vi "Camer Control Main.vi"() -> ()   [LabVIEW 2014]
uses:
  <vilib>/MakerHub/LINX/Public/Utilities/Open Local.vi
  FGV/Camer Control Variables.vi
  Application Support/Stop Button/SubVI/Get Stop Button Status.vi
  Aircraft Information/Sub VI/Get Aircraft Information.vi
  <vilib>/MakerHub/LINX/LMH-LINX.lvlib
panel:
  out "Device Name":string
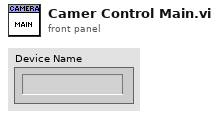
[diagram p1: front panel]
types:
  T1 = typedef "LMH-LINX.lvlib/LINX Ref.ctl" = cluster{"IO":T2, "Interface":T3, "LINX Device Config":T4}
  T2 = typedef "LMH-LINX.lvlib/Platform.ctl" = enum16{"Remote", "Local"}
  T3 = typedef "LMH-LINX.lvlib/Interface.ctl" = enum16{"Serial", "TCP"}
  T4 = typedef "LMH-LINX.lvlib/Device.lvlib/LINX Device Config.ctl" = cluster{"Interface":T3, "COM Port":refnum<visa-resource-name>, "TCP Configuration":T5, "Device Family":u8, "Device ID":u8, "Device Name":string, "TCP Ref":refnum<k5>, "Channels":T6}
  T5 = typedef "LMH-LINX.lvlib/Device.lvlib/TCP Config.ctl" = cluster{"IP Address":string, "Port":u16}
  T6 = typedef "LMH-LINX.lvlib/Channels.ctl" = cluster{"DI":u8[], "DO":u8[], "AI":u8[], "AO":u8[], "PWM":u8[], "QE":u8[], "UART":u8[], "I2C 2":u8[], "SPI":u8[], "CAN":u8[], "Servo":u8[], "AI Ref (V)":dbl, "AI Resolution (Bits)":u8, "AO Ref (V)":dbl, "AO Resolution (Bits)":u8}
  T7 = typedef "Drone Information.ctl" = cluster{"Aircraft ID":u8, "Tag ID":string, "System Status":string, "Base Mode":T8, "Armed/Disarmed":bool, "Battery Voltage":dbl, "Control Mode":T9, "Initialisation":u8, "Coms with aircraft good":bool, "Mode":string, "Mission Uploaded":bool}
  T8 = typedef "Base Mode.ctl" = cluster{"Custom Mode":bool, "Test Enabled":bool, "Autonomous Mode":bool, "Guided Mode":bool, "Stabilization Enabled":bool, "HIL Enabled":bool, "Manual Mode":bool, "Arm":bool}
  T9 = typedef "Aircraft Mode.ctl" = enum16{"Loiter", "Stabalise", "Failsafe", "Emergency Stop"}
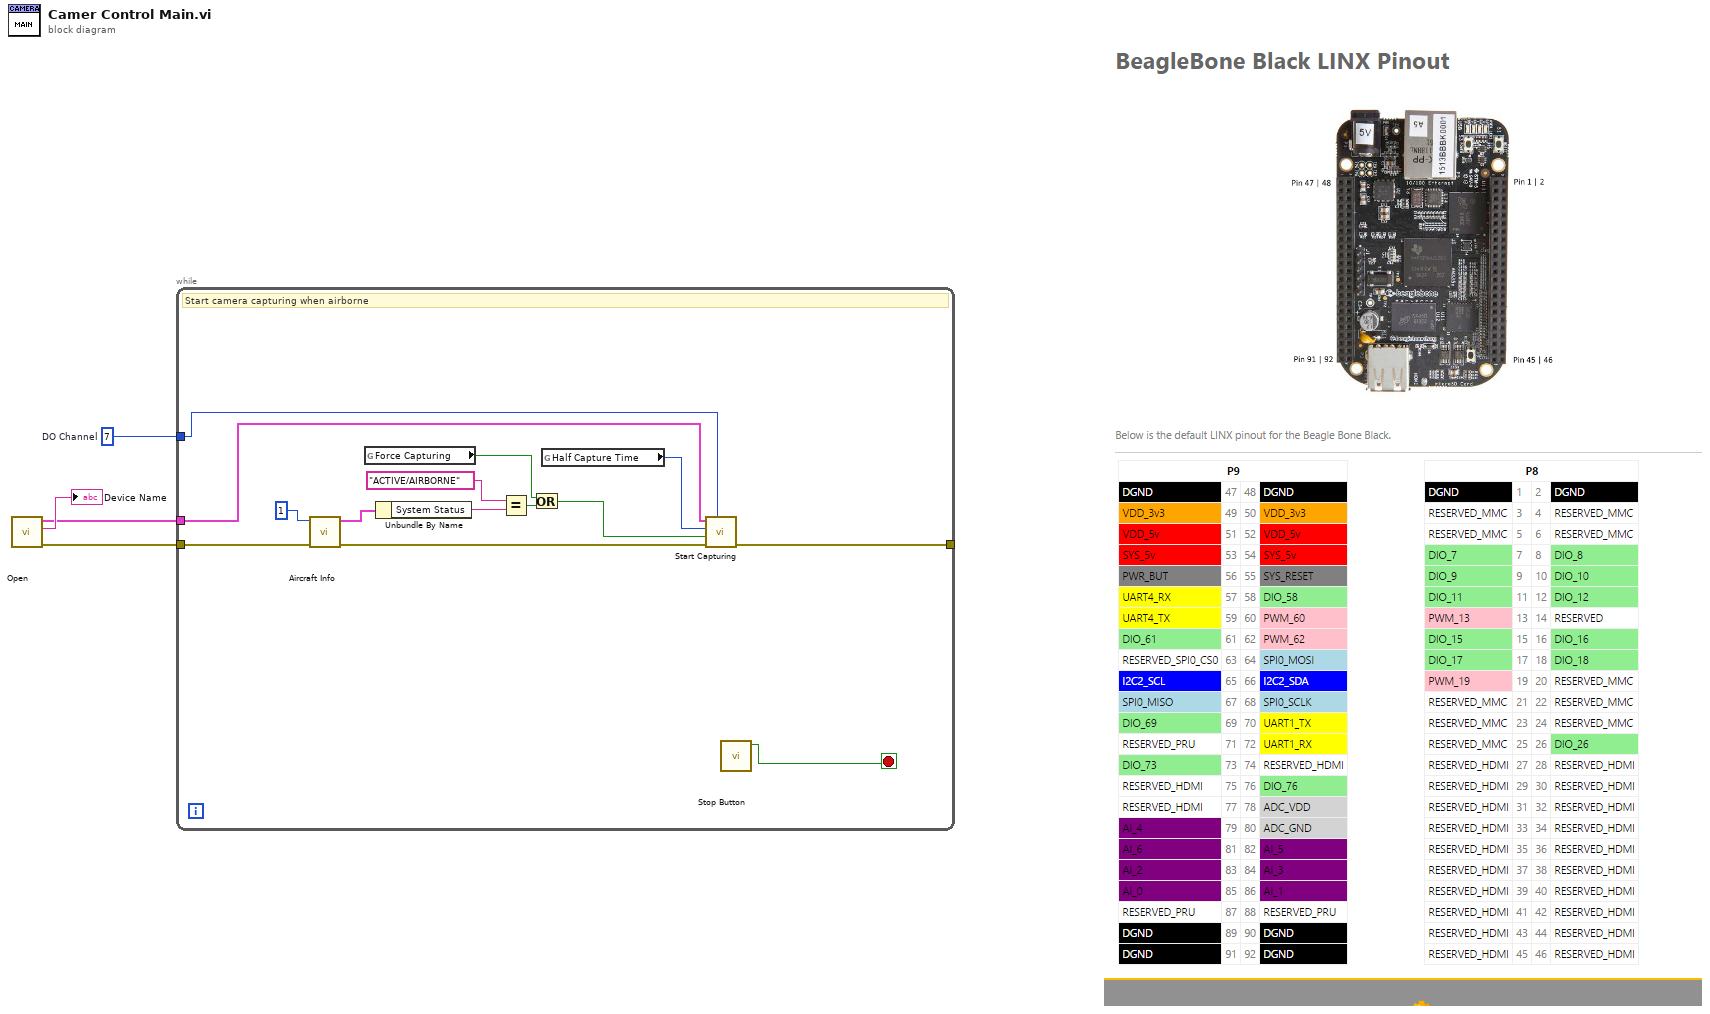
[diagram p0: block diagram]
diagram:
  w1 = u8 7  # DO Channel
  n1 = call-poly <vilib>:"Open.vi"() -> ("Error Out"=w3:errorcluster, "Device Name"=→"Device Name":string, "LINX Resource"=w2:T1)  [unwired: 9 in]
  n2 = while {
    tunnel: w3 -> [w18]
    tunnel: w2 -> [w6]
    tunnel: w1 -> [w5]
    tunnel: [w8] -> _
    stop <- w11 stop-if-true
    # "Start camera capturing when airborne"
    n3 = call-poly "Aircraft Info.vi"("Error In"=w18, "Aircraft ID"=u8 1) -> ("Error Out"=w10:errorcluster, "Aircraft Information Out"=w16:T7)  [unwired: 8 in]
    n4 = global read "Camer Control Variables.vi" "Force Capturing"() -> (w12:bool)
    n5 = Unbundle By Name(w16) -> ("System Status"=w15:string)
    n6 = Equal?(x="ACTIVE/AIRBORNE", y=w15) -> (x = y?=w13:bool)
    n7 = Or(x=w12, y=w13) -> (x .or. y?=w9:bool)
    n8 = global read "Camer Control Variables.vi" "Half Capture Time"() -> (w7:u32)
    n9 = call "Start Capturing.vi"("DO Channel"=w5, "Error In"=w10, "Start Capture"=w9, "Half capture time"=w7, "LINX Resource"=w6) -> ("Error Out"=w8:errorcluster)  [unwired: 5 in, 1 out]
    n10 = call-poly "Stop Button.vi"() -> ("Stop ButtonOut"=w11:bool)  [unwired: 10 in, 1 out]
  }
